vi "terminate.vi"(8 "error in (no error)":errorcluster, 11 "SignalReaderDL091205FPGA in":refnum<class "SignalReaderDL091205FPGA.lvclass">) -> (0 "error out":errorcluster, 3 "SignalReaderDL091205FPGA out":refnum<class "SignalReaderDL091205FPGA.lvclass">)   [LabVIEW 2010, in "SignalReaderDL091205FPGA.lvclass"]
doc: "The dynamic dispatch version of this VI terminates the plug-in object by releasing all of its resources."
uses:
  SignalReaderDL091205FPGA.lvclass
  SignalReaderDL091205FPGA.lvclass/SignalReaderDL091205FPGA.ctl
  FPGAWrapper/GenericFPGAWrapper/GenericFPGAWrapper/GenericFPGAWrapper.lvclass
  GenericSignalReader/GenericSignalReader/GenericSignalReader.lvclass
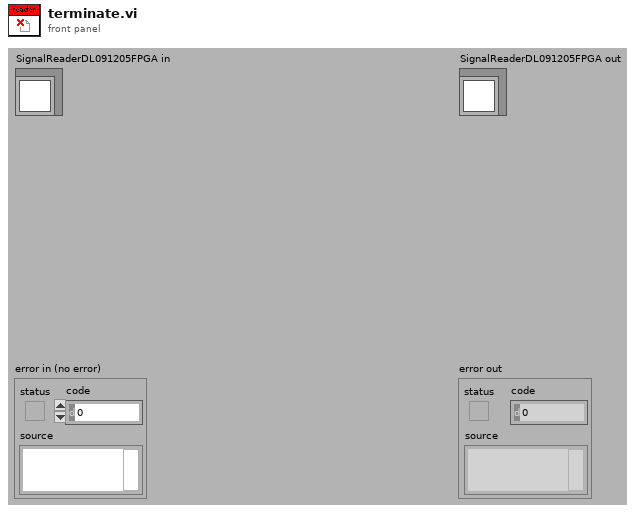
[diagram p1: front panel]
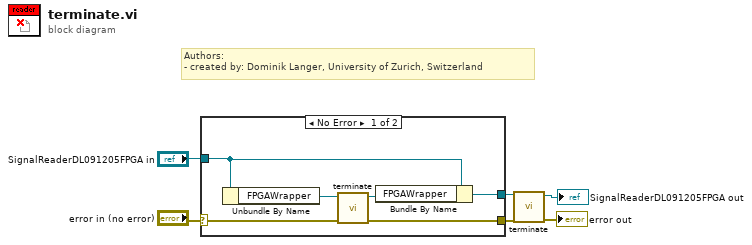
[diagram p0: block diagram]
diagram:
  # "Authors: \n- created by: Dominik Langer, University of Zurich, Switzerland"
  n1 = case shown="No Error" "error in (no error)" {
    selector: "error in (no error)" -> [w7 w14]
    tunnel: [w8 w14] -> w4
    tunnel: [w12 w13] -> w3
    tunnel: "SignalReaderDL091205FPGA in" -> [w11 w13]
    frame No Error {
      n2 = Unbundle By Name(w11) -> ("FPGAWrapper"=w10:refnum<class "GenericFPGAWrapper.lvclass">)
      n3 = call-dynamic "terminate.vi"("error in (no error)"=w7, "GenericPlugin in"=w10) -> ("error out"=w8:errorcluster, "GenericPlugin out"=w9:refnum<class "GenericFPGAWrapper.lvclass">)  [unwired: 8 out]
      n4 = Bundle By Name(cluster=w11, "FPGAWrapper"=w9) -> (w12:refnum<class "SignalReaderDL091205FPGA.lvclass">)
    }
    frame Error {
    }
  }
  n5 = call-parent "terminate.vi"("error in (no error)"=w4, "GenericPlugin in"=w3) -> ("error out"=→"error out":errorcluster, "GenericPlugin out"=→"SignalReaderDL091205FPGA out":refnum<class "SignalReaderDL091205FPGA.lvclass">)  [unwired: 8 in]
